vi "expandInputParams.vi"(10 "Profilometry?":bool, 11 "Frequencies":dbl[](array[numeric])) -> (0 "Number Images":dbl, 1 "Orientation Vector":bool[](array[boolean]), 2 "Phase Vector":dbl[](array[numeric]), 3 "Frequency Vector":dbl[](array[numeric]))   [LabVIEW 2017]
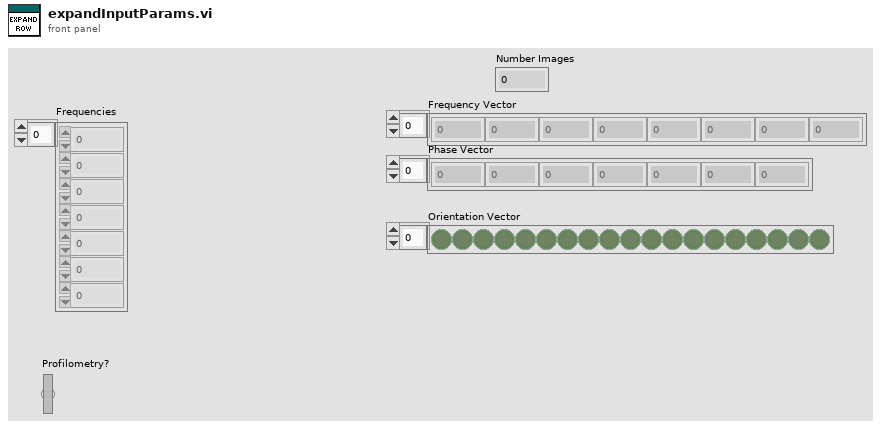
[diagram p1: front panel]
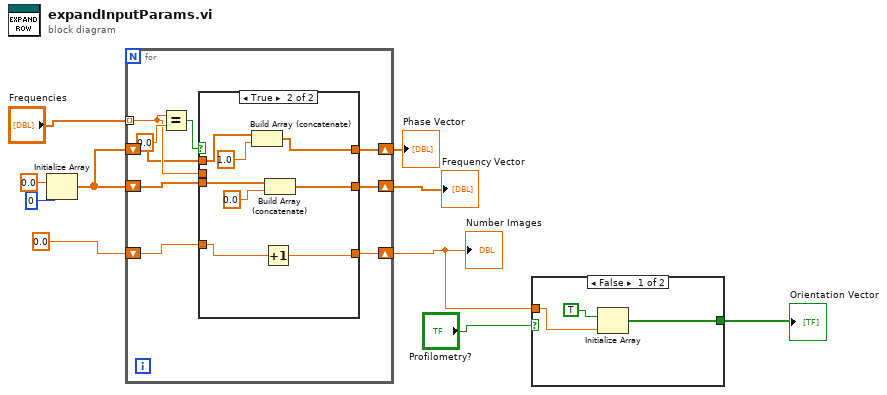
[diagram p0: block diagram]
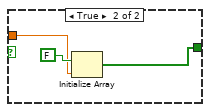
[diagram p2: hidden frame]
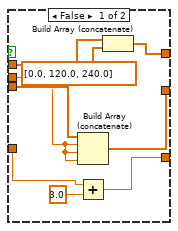
[diagram p3: hidden frame]
diagram:
  n1 = Initialize Array(0.0 ("element"), 0 ("dimension size")) -> (w5:dbl[])
  n2 = for {
    tunnel: "Frequencies" -> [w13] mode=indexing
    shift-right: [w17] -> w2
    shift-left: 0.0 -> [w16]
    shift-right: [w15] -> w9
    shift-left: w5 -> [w14]
    shift-right: [w12] -> w4
    shift-left: w5 -> [w11]
    n3 = Equal?(x=w13, y=0.0) -> (x = y?=w19:bool)
    n4 = case shown="True" w19 {
      tunnel: [w27 w35] -> w17
      tunnel: w16 -> [w26 w36]
      tunnel: [w24 w34] -> w15
      tunnel: w14 -> [w25 w33]
      tunnel: w13 -> [w23 _]
      tunnel: [w22 w30] -> w12
      tunnel: w11 -> [w21 w31]
      frame False {
        n5 = Build Array (concatenate)(w25, w23, w23, w23) -> (w24:dbl[])
        n6 = Add(x=w26, y=3.0) -> (x+y=w27:dbl)
        n7 = Build Array (concatenate)(w21, dbl[] [0.0, 120.0, 240.0] ("array")) -> (w22:dbl[])
      }
      frame True {
        n8 = Build Array (concatenate)(w31, 1.0) -> (w30:dbl[])
        n9 = Increment(x=w36) -> (x+1=w35:dbl)
        n10 = Build Array (concatenate)(w33, 0.0) -> (w34:dbl[])
      }
    }
  }
  "Number Images" <- w2
  "Frequency Vector" <- w9
  "Phase Vector" <- w4
  n11 = case shown="False" "Profilometry?" {
    tunnel: w2 -> [w39 w41]
    tunnel: [w37 w40] -> w1
    frame False {
      n12 = Initialize Array(TRUE, w39) -> (w37:bool[])
    }
    frame True {
      n13 = Initialize Array(FALSE, w41) -> (w40:bool[])
    }
  }
  "Orientation Vector" <- w1
